vi "Dispose.vi"(8 "error in (no error)":errorcluster, 11 "Test Executor in":refnum<class "Test Executor.lvclass">) -> (0 "error out":errorcluster, 2 "Result Queue":refnum<queue>, 3 "Application":refnum<vi>)   [LabVIEW 2017, in "Test Executor.lvclass"]
uses:
  Test Executor.lvclass
  Test Result/Test Result.lvclass
  Test Executor.lvclass/Test Executor.ctl
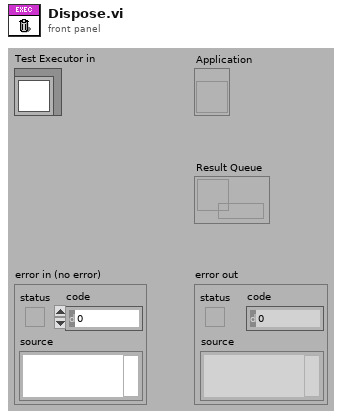
[diagram p1: front panel]
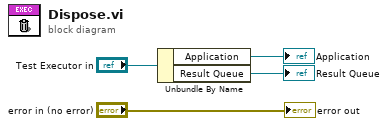
[diagram p0: block diagram]
diagram:
  n1 = Unbundle By Name("Test Executor in") -> ("Application"=→"Application":refnum<vi>, "Result Queue"=→"Result Queue":refnum<queue>)
  "error out" <- "error in (no error)"
